vi "ex1.vi"() -> ()   [LabVIEW 2022 SP3]
uses:
  <vilib>/numeric/Random Number (Range) I64.vi
  7e490bf8-fc35-4ee5-afc7-ebb8f6895de7.vi
  541270c6-a71e-4034-9e51-2e389e5b9272.vi
  <vilib>/numeric/sub_Random U32.vi
  <vilib>/Array/Sort 2D Array - Pop Stack.vi
  <vilib>/Array/Sort 2D Array - Push Stack.vi
  7e490bf8-fc35-4ee5-afc7-ebb8f6895de7.vi/269d4b3b-47f5-49e3-8884-44851e4dd9d5.vi
  7e490bf8-fc35-4ee5-afc7-ebb8f6895de7.vi/6d99389c-673d-4efb-bf33-19b32bcf4cf8.vi
  541270c6-a71e-4034-9e51-2e389e5b9272.vi/269d4b3b-47f5-49e3-8884-44851e4dd9d5.vi
  541270c6-a71e-4034-9e51-2e389e5b9272.vi/6d99389c-673d-4efb-bf33-19b32bcf4cf8.vi
panel:
  in  "Sort By:":enum16{"column", "row"}(ring)
  in  "Select Row":dbl
  in  "Select Column":dbl
  out "Output Array":i64[][](array[numeric])
  in  "Dimension Size":i32
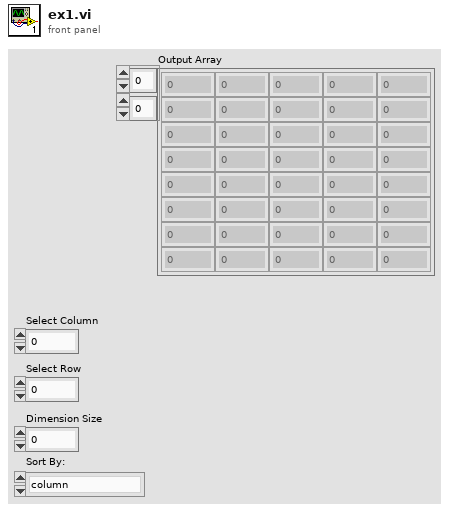
[diagram p1: front panel]
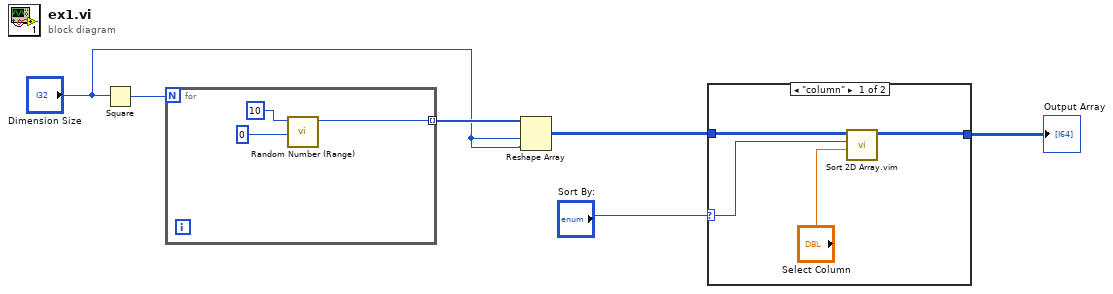
[diagram p0: block diagram]
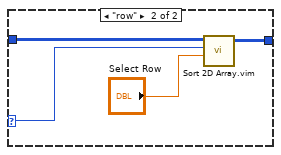
[diagram p2: hidden frame]
diagram:
  n1 = Square(x="Dimension Size") -> (x^2=w4:i32)
  n2 = for {
    N: w4 -> [_]
    tunnel: [w9] -> w6 mode=indexing
    n3 = call-poly <vilib>:"Random Number (Range).vi"("lower bound (-100)"=i64 0, "upper bound (100)"=i64 10) -> ("number"=w9:i64)  [unwired: 9 in]
  }
  n4 = Reshape Array(w6, "Dimension Size", "Dimension Size") -> (w3:i64[][])
  n5 = case shown="\"column\"" "Sort By:" {
    selector: "Sort By:" -> [w10 w14]
    tunnel: w3 -> [w13 w17]
    tunnel: [w12 w16] -> w2
    frame "column" {
      n6 = call "Sort 2D Array.vim"("index"="Select Column", "dimension to index (column)"=w10, "2D array"=w13) -> ("sorted 2D array"=w12:i64[][])  [unwired: 7 in, 1 out]
    }
    frame "row" {
      n7 = call "Sort 2D Array.vim"("index"="Select Row", "dimension to index (column)"=w14, "2D array"=w17) -> ("sorted 2D array"=w16:i64[][])  [unwired: 7 in, 1 out]
    }
  }
  "Output Array" <- w2
